vi "Assert cal Attendance.vi"() -> ()   [LabVIEW 2015, in "Admin_Actor.lvlib" / "MemberAttendance.lvclass"]
uses:
  MemberAttendance.lvclass
  ExcelReader/ExcelReader.lvclass
panel:
  out "Attendance Result(\"\")":string[][](array[string])
  in  "Path":path
  in  "ExcelReader in":refnum<class "ExcelReader.lvclass">
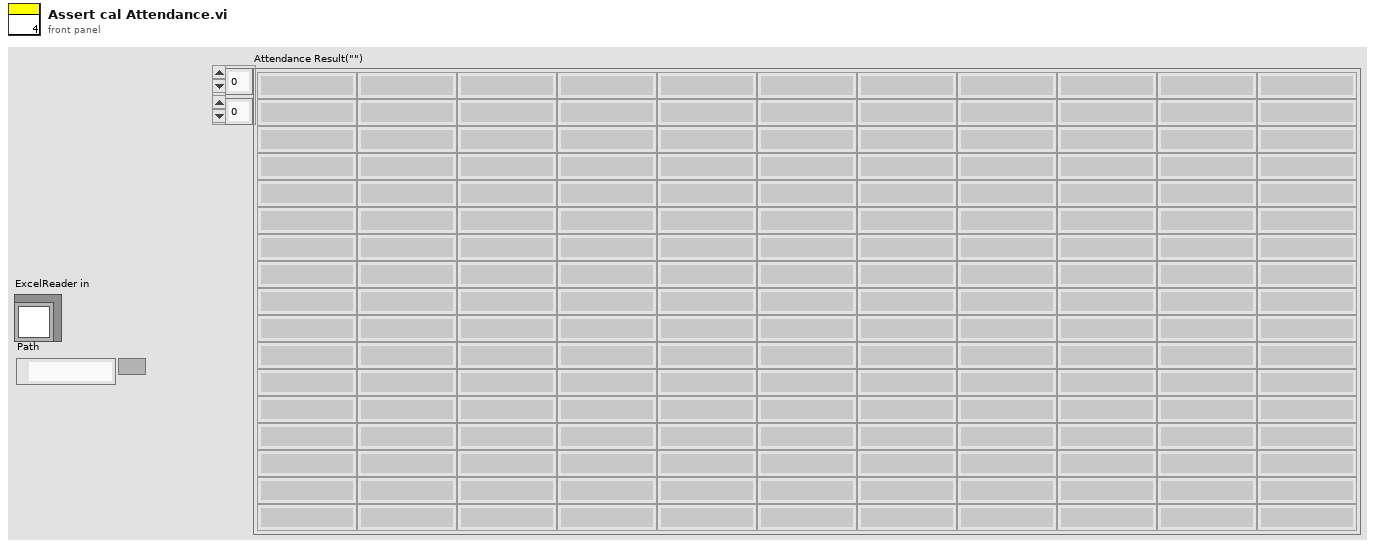
[diagram p1: front panel]
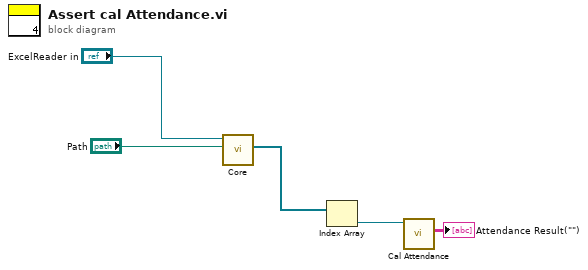
[diagram p0: block diagram]
diagram:
  n1 = call "Core.vi"("Path"="Path", "ExcelReader in"="ExcelReader in") -> ("MemberAttendance"=w3:refnum<class "MemberAttendance.lvclass">[])  [unwired: 7 in, 2 out]
  n2 = Index Array(array=w3) -> (element=w2:refnum<class "MemberAttendance.lvclass">)  [unwired: 1 in]
  n3 = call "Cal Attendance.vi"("MemberAttendance in"=w2) -> ("Attendance Result(\"\")"=→"Attendance Result(\"\")":string[][])  [unwired: 8 in, 2 out]
